vi "Open Log Files.vi"() -> (0 "error out":errorcluster, 2 "drive log":refnum<file>, 3 "copilot log":refnum<file>)   [LabVIEW 2014]
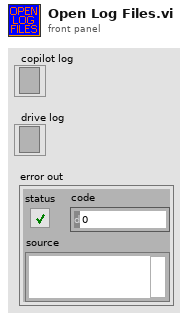
[diagram p1: front panel]
types:
  T1 = enum16{"open", "replace", "create", "open or create", "replace or create", "replace or create with confirmation"}
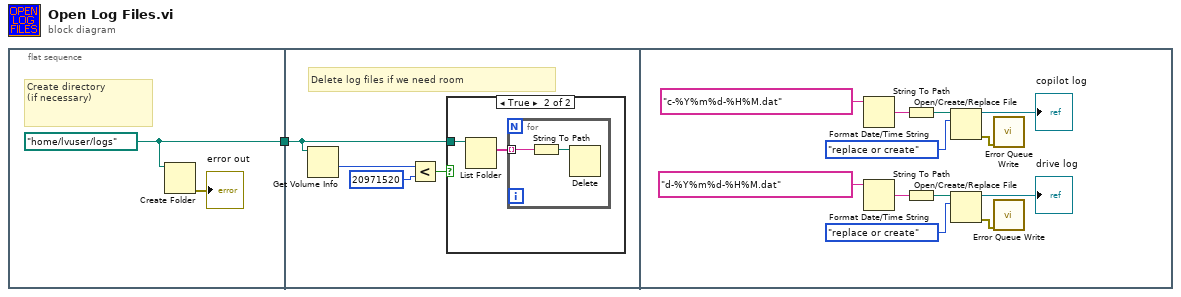
[diagram p0: block diagram]
diagram:
  n1 = flat-sequence {
    tunnel: [w3] -> w1
    tunnel: w1 -> [w4]
    frame #0 {
      w3 = path "/home/lvuser/logs" ("path (use dialog)")
      # "Create directory\n(if necessary)"
      n2 = Create Folder(path (use dialog)=w3) -> (error out=→"error out":errorcluster)  [unwired: 2 in, 2 out]
    }
    frame #1 {
      # "Delete log files if we need room"
      n3 = Get Volume Info(11:w4) -> (1:w7:i64)  [unwired: 1 in, 5 out]
      n4 = Less?(x=w7, y=i64 20971520) -> (x < y?=w5:bool)
      n5 = case shown="True" w5 {
        tunnel: w4 -> [_ w8]
        frame False {
        }
        frame True {
          n6 = List Folder(path=w8) -> (filenames=w9:string[])  [unwired: 3 in, 3 out]
          n7 = for {
            tunnel: w9 -> [w10] mode=indexing
            n8 = String To Path(string=w10) -> (path=w11:path)
            n9 = Delete(path (use dialog)=w11) -> ()  [unwired: 4 in, 3 out]
          }
        }
      }
    }
    frame #2 {
      n10 = Format Date/Time String(time format string (%c)="c-%Y%m%d-%H%M.dat") -> (date/time string=w17:string)  [unwired: 2 in]
      n11 = Format Date/Time String(time format string (%c)="d-%Y%m%d-%H%M.dat") -> (date/time string=w12:string)  [unwired: 2 in]
      n12 = String To Path(string=w17) -> (path=w18:path)
      n13 = String To Path(string=w12) -> (path=w13:path)
      n14 = Open/Create/Replace File(file path (use dialog)=w18, operation (0:open)=T1."replace or create") -> (refnum out=→"copilot log":refnum<file>, error out=w19:errorcluster)  [unwired: 4 in, 1 out]
      n15 = Open/Create/Replace File(file path (use dialog)=w13, operation (0:open)=T1."replace or create") -> (refnum out=→"drive log":refnum<file>, error out=w16:errorcluster)  [unwired: 4 in, 1 out]
      n16 = call "Error Queue Write.vi"("error in (no error)"=w19) -> ()  [unwired: 11 in]
      n17 = call "Error Queue Write.vi"("error in (no error)"=w16) -> ()  [unwired: 11 in]
    }
  }
